vi "Extreme Value CDF.vi"(9 "b":dbl=1.0, 10 "a":dbl, 11 "x":dbl) -> (0 "error":i32, 3 "cdf(x)":dbl=0.6321205588285577)   [LabVIEW 2018, in "NI_Gmath.lvlib"]
doc: "Computes the continuous cumulative distribution function (CDF), or the probability that the random variate X, where X describes the selected distribution type, has a value less than or equal to <B>x</B>. You must manually select the polymorphic instance to use."
uses:
  NI_Gmath.lvlib
  st_error_code.ctl
panel:
  # "Extreme Value CDF"
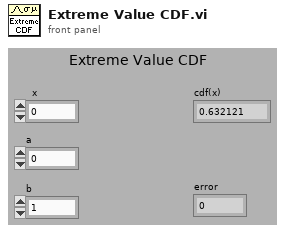
[diagram p1: front panel]
types:
  T1 = typedef "NI_Gmath.lvlib/st_error_code.ctl" = i32
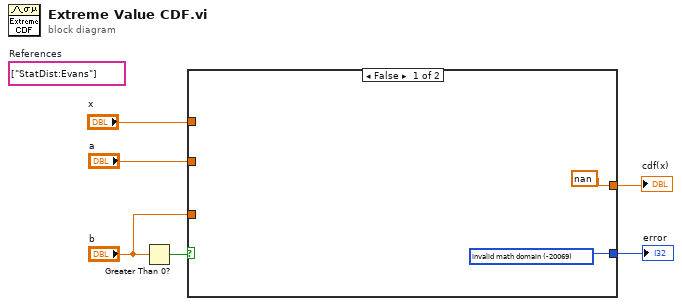
[diagram p0: block diagram]
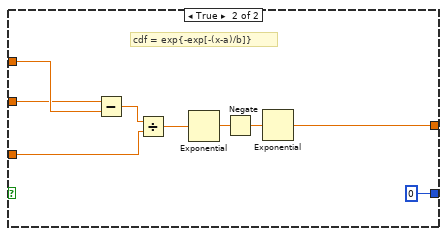
[diagram p2: hidden frame]
diagram:
  (unwired) string[] ["StatDist:Evans"]  # References
  n1 = Greater Than 0?(x="b") -> (x > 0?=w3:bool)
  n2 = case shown="False" w3 {
    tunnel: "b" -> [_ w12]
    tunnel: [w7 0 ("invalid math domain")] -> w1
    tunnel: [nan w9] -> w2
    tunnel: "x" -> [_ w16]
    tunnel: "a" -> [_ w15]
    frame False {
      w7 = T1 -20069 items=["invalid math domain"=-20069, "Fourier interpolation size m >= n"=-20070, "empty array"=-20003] ("stat interp error code")
    }
    frame True {
      # "cdf = exp{-exp[-(x-a)/b]}"
      n3 = Subtract(x=w15, y=w16) -> (x-y=w14:dbl)
      n4 = Divide(x=w14, y=w12) -> (x/y=w10:dbl)
      n5 = Exponential(1:w10) -> (0:w11:dbl)
      n6 = Negate(x=w11) -> (-x=w13:dbl)
      n7 = Exponential(1:w13) -> (0:w9:dbl)
    }
  }
  "cdf(x)" <- w2
  "error" <- w1
